vi "TL_Driver.vi"(0 "Device In":refnum<visa-resource-name>="Pro8000", 5 "Commands":T1(ring)=enum."SET", 7 "Settings":T3={"Module"=enum."Off Line TEC", "OnLineTEC"=23.2280006, "OnLineLD"=0.1722, "OffLineTEC"=29.538, "OffLineLD"=0.173, "EtalonTEC"=27.0004501, "TSOA-TEC"=18.9999638} {"OffLineLD" min=0.0 max=0.18 step=0.001 format="%.3p"; "OnLineLD" min=0.0 max=0.18 step=0.001 format="%.3p"; "TSOA-TEC" format="%.2g"; "EtalonTEC" format="%.2g"; "OffLineTEC" min=16.0 max=30.0 step=0.1 format="%.3g"; "OnLineTEC" min=16.0 max=28.0 step=0.1 format="%.3g"}, 11 "error in":errorcluster) -> (4 "Device Out":refnum<visa-resource-name>="Pro8000", 6 "Response":string, 8 "Readings":T2={"OnLineTEC"=23.2342777, "OnLineLD"=0.172234386, "OffLineTEC"=29.5498905, "OffLineLD"=0.17301172, "EtalonTEC"=27.0301247, "TSOA-TEC"=19.0111637, "Pro8000"=TRUE, "OnLine TEC"=TRUE, "OnLine LD"=TRUE, "OffLine TEC"=TRUE, "OffLine LD"=TRUE, "Etalon TEC"=TRUE, "TSOA TEC"=TRUE} {"OffLineLD" format="%.3p"; "OnLineLD" format="%.3p"; "TSOA-TEC" format="%.3g"; "EtalonTEC" format="%.3g"; "OffLineTEC" format="%.3g"; "OnLineTEC" format="%.3g"}, 15 "error out":errorcluster)   [LabVIEW 2012]
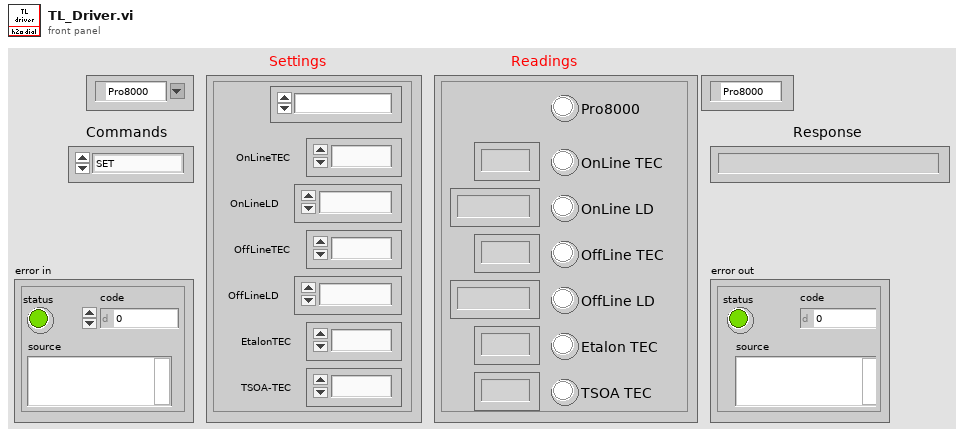
[diagram p1: front panel]
types:
  T1 = enum16{"Open_TL", "Close_TL", "Verify_ID", "TEC_Sensor", "SET", "READ", "ON", "OFF", "Set_Limits", "Read_Limits", "Enable_Status", "Read_Status"}
  T2 = cluster{"OnLineTEC":dbl, "OnLineLD":dbl, "OffLineTEC":dbl, "OffLineLD":dbl, "EtalonTEC":dbl, "TSOA-TEC":dbl, "Pro8000":bool, "OnLine TEC":bool, "OnLine LD":bool, "OffLine TEC":bool, "OffLine LD":bool, "Etalon TEC":bool, "TSOA TEC":bool}
  T3 = cluster{"Module":enum16{"On Line TEC", "On Line LD", "Off Line TEC", "Off Line LD", "Etalon TEC", "TSOA TEC"}, "OnLineTEC":dbl, "OnLineLD":dbl, "OffLineTEC":dbl, "OffLineLD":dbl, "EtalonTEC":dbl, "TSOA-TEC":dbl}
  T4 = enum16{"On Line TEC", "On Line LD", "Off Line TEC", "Off Line LD", "Etalon TEC", "TSOA TEC"}
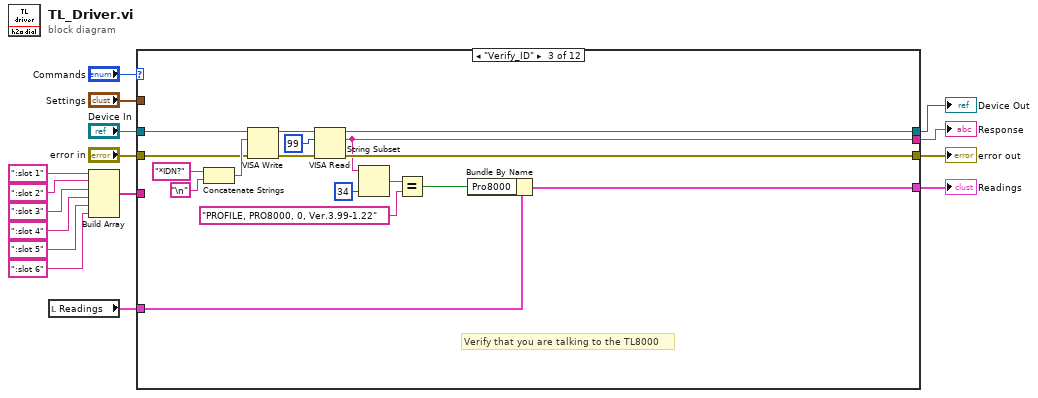
[diagram p0: block diagram]
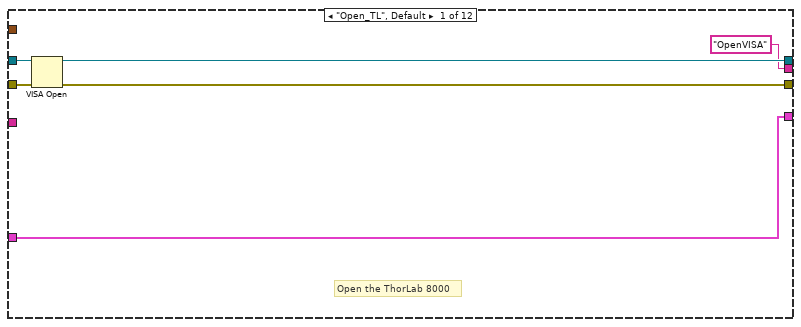
[diagram p2: hidden frame]
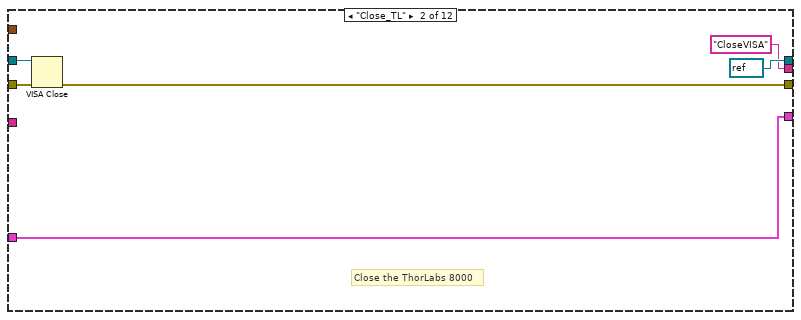
[diagram p3: hidden frame]
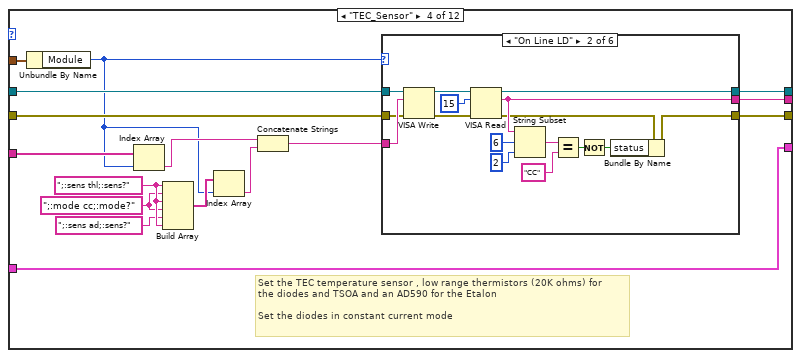
[diagram p4: hidden frame]
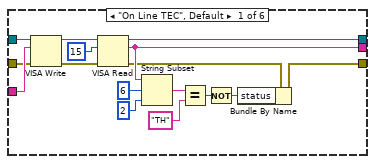
[diagram p5: hidden frame]
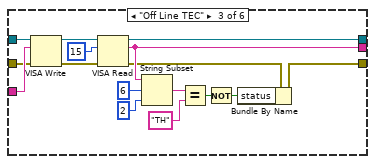
[diagram p6: hidden frame]
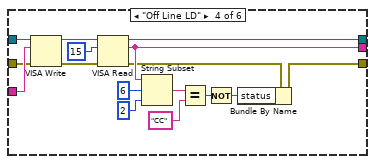
[diagram p7: hidden frame]
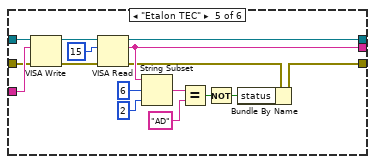
[diagram p8: hidden frame]
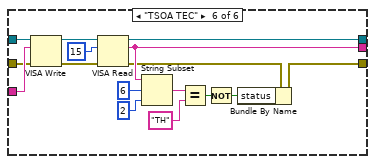
[diagram p9: hidden frame]
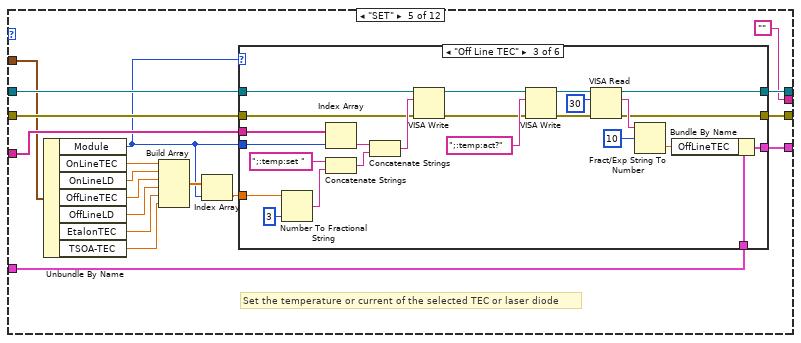
[diagram p10: hidden frame]
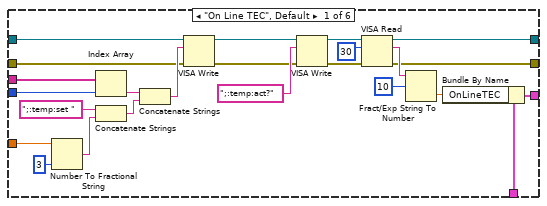
[diagram p11: hidden frame]
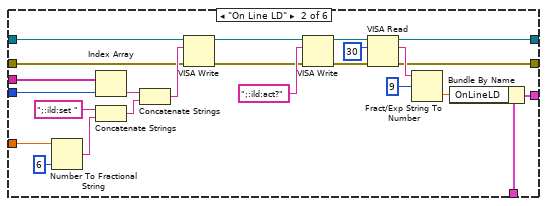
[diagram p12: hidden frame]
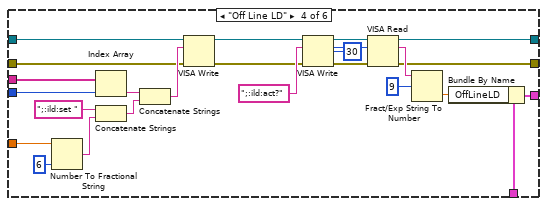
[diagram p13: hidden frame]
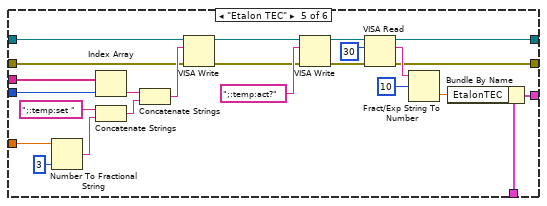
[diagram p14: hidden frame]
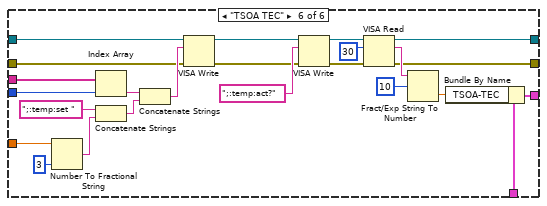
[diagram p15: hidden frame]
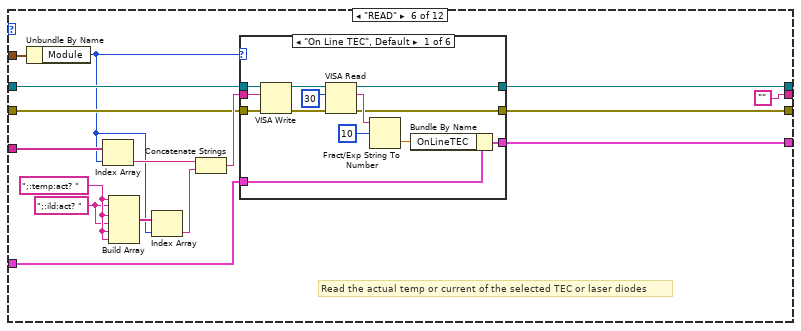
[diagram p16: hidden frame]
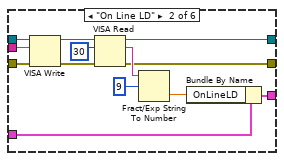
[diagram p17: hidden frame]
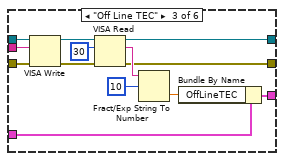
[diagram p18: hidden frame]
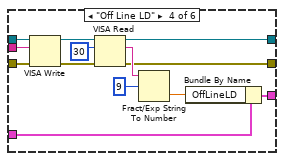
[diagram p19: hidden frame]
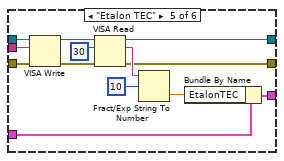
[diagram p20: hidden frame]
diagram:
  n1 = local read "Readings"() -> (w2:T2)
  n2 = Build Array(":slot 1", ":slot 2", ":slot 3", ":slot 4", ":slot 5", ":slot 6") -> (w13:string[])
  n3 = case shown="\"Verify_ID\"" "Commands" {
    tunnel: "Device In" -> [w22 w28 w42 w60 w175 w334 w428 w552 w668 w672 w676 w683]
    tunnel: "error in" -> [w21 w27 w39 w59 w174 w333 w427 w551 w669 w673 w677 w686]
    tunnel: [w20 refnum<visa-resource-name> refnum ("VISA resource name") w37 w58 w171 w329 w424 w548 w668 w672 w676 w684] -> w11
    tunnel: [w19 w26 w36 w55 w172 w328 w423 w547 w669 w673 w677 w682] -> w15
    tunnel: ["OpenVISA" "CloseVISA" w35 w57 "" "" w422 w546 "" "" "" "Read Status"] -> w10
    tunnel: w13 -> [_ _ _ w54 w173 w331 w425 w549 _ _ _ w687]
    tunnel: "Settings" -> [_ _ _ w53 w169 w327 w421 w545 _ _ _ w685]
    tunnel: w2 -> [w17 w23 w31 w47 w159 w326 w420 w544 w670 w674 w678 w681]
    tunnel: [w17 w23 w30 w47 w158 w325 w419 w543 w670 w674 w678 w680] -> w1
    frame "Open_TL", Default {
      # "Open the ThorLab 8000"
      n4 = VISA Open(error in (no error)=w21, VISA resource name=w22) -> (VISA resource name=w20:refnum<visa-resource-name>, error out=w19:errorcluster)  [unwired: 3 in]
    }
    frame "Close_TL" {
      # "Close the ThorLabs 8000"
      n5 = VISA Close(VISA resource name=w28, error in (no error)=w27) -> (error out=w26:errorcluster)
    }
    frame "Verify_ID" {
      # "Verify that you are talking to the TL8000"
      n6 = Concatenate Strings("*IDN?" ("string"), "\n") -> (w43:string)
      n7 = VISA Write(VISA resource name=w42, write buffer=w43, error in (no error)=w39) -> (VISA resource name out=w40:refnum<visa-resource-name>, error out=w38:errorcluster)  [unwired: 1 out]
      n8 = VISA Read(VISA resource name=w40, byte count=u32 99, error in (no error)=w38) -> (VISA resource name out=w37:refnum<visa-resource-name>, read buffer=w35:string, error out=w36:errorcluster)  [unwired: 1 out]
      n9 = String Subset(string=w35, length (rest)=34 ("length (rest)")) -> (substring=w33:string)  [unwired: 1 in]
      n10 = Equal?(x=w33, y="PROFILE, PRO8000, 0, Ver.3.99-1.22" ("Response")) -> (x = y?=w29:bool)
      n11 = Bundle By Name(cluster=w31, "Pro8000"=w29) -> (w30:T2)
    }
    frame "TEC_Sensor" {
      w46 = ";:mode cc;:mode?"
      w52 = ";:sens thl;:sens?" ("string")
      # "Set the TEC temperature sensor , low range thermistors (20K ohms) for\nthe diodes and TSOA and an AD590 for the Etalon\n\nSet the diodes in constant current mode"
      n12 = Unbundle By Name(w53) -> ("Module"=w48:T4)
      n13 = Index Array(array=w54, index=w48) -> (element=w56:string)
      n14 = Build Array(w52, w46, w52, w46, ";:sens ad;:sens?" ("string"), w52) -> (w49:string[])
      n15 = Index Array(array=w49, index=w48) -> (element=w50:string)
      n16 = Concatenate Strings(w56, w50) -> (w61:string)
      n17 = case shown="\"On Line LD\"" w48 {
        tunnel: w61 -> [w77 w93 w109 w125 w141 w157]
        tunnel: w60 -> [w76 w92 w108 w124 w140 w156]
        tunnel: w59 -> [w75 w91 w107 w123 w139 w155]
        tunnel: [w74 w90 w106 w122 w138 w154] -> w58
        tunnel: [w73 w89 w105 w121 w137 w153] -> w57
        tunnel: [w72 w88 w104 w120 w136 w152] -> w55
        frame "On Line TEC", Default {
          n18 = VISA Write(VISA resource name=w76, write buffer=w77, error in (no error)=w75) -> (VISA resource name out=w64:refnum<visa-resource-name>, error out=w63:errorcluster)  [unwired: 1 out]
          n19 = VISA Read(VISA resource name=w64, byte count=u32 15, error in (no error)=w63) -> (VISA resource name out=w74:refnum<visa-resource-name>, read buffer=w73:string, error out=w70:errorcluster)  [unwired: 1 out]
          n20 = String Subset(string=w73, offset (0)=6 ("length (rest)"), length (rest)=2 ("length (rest)")) -> (substring=w67:string)
          n21 = Equal?(x=w67, y="TH") -> (x = y?=w66:bool)
          n22 = Not(x=w66) -> (.not. x?=w65:bool)
          n23 = Bundle By Name(cluster=w70, "status"=w65) -> (w72:errorcluster)
        }
        frame "On Line LD" {
          n24 = VISA Write(VISA resource name=w92, write buffer=w93, error in (no error)=w91) -> (VISA resource name out=w80:refnum<visa-resource-name>, error out=w79:errorcluster)  [unwired: 1 out]
          n25 = VISA Read(VISA resource name=w80, byte count=u32 15, error in (no error)=w79) -> (VISA resource name out=w90:refnum<visa-resource-name>, read buffer=w89:string, error out=w86:errorcluster)  [unwired: 1 out]
          n26 = String Subset(string=w89, offset (0)=6 ("length (rest)"), length (rest)=2 ("length (rest)")) -> (substring=w83:string)
          n27 = Equal?(x=w83, y="CC") -> (x = y?=w82:bool)
          n28 = Not(x=w82) -> (.not. x?=w81:bool)
          n29 = Bundle By Name(cluster=w86, "status"=w81) -> (w88:errorcluster)
        }
        frame "Off Line TEC" {
          n30 = VISA Write(VISA resource name=w108, write buffer=w109, error in (no error)=w107) -> (VISA resource name out=w96:refnum<visa-resource-name>, error out=w95:errorcluster)  [unwired: 1 out]
          n31 = VISA Read(VISA resource name=w96, byte count=u32 15, error in (no error)=w95) -> (VISA resource name out=w106:refnum<visa-resource-name>, read buffer=w105:string, error out=w102:errorcluster)  [unwired: 1 out]
          n32 = String Subset(string=w105, offset (0)=6 ("length (rest)"), length (rest)=2 ("length (rest)")) -> (substring=w99:string)
          n33 = Equal?(x=w99, y="TH") -> (x = y?=w98:bool)
          n34 = Not(x=w98) -> (.not. x?=w97:bool)
          n35 = Bundle By Name(cluster=w102, "status"=w97) -> (w104:errorcluster)
        }
        frame "Off Line LD" {
          n36 = VISA Write(VISA resource name=w124, write buffer=w125, error in (no error)=w123) -> (VISA resource name out=w112:refnum<visa-resource-name>, error out=w111:errorcluster)  [unwired: 1 out]
          n37 = VISA Read(VISA resource name=w112, byte count=u32 15, error in (no error)=w111) -> (VISA resource name out=w122:refnum<visa-resource-name>, read buffer=w121:string, error out=w118:errorcluster)  [unwired: 1 out]
          n38 = String Subset(string=w121, offset (0)=6 ("length (rest)"), length (rest)=2 ("length (rest)")) -> (substring=w115:string)
          n39 = Equal?(x=w115, y="CC") -> (x = y?=w114:bool)
          n40 = Not(x=w114) -> (.not. x?=w113:bool)
          n41 = Bundle By Name(cluster=w118, "status"=w113) -> (w120:errorcluster)
        }
        frame "Etalon TEC" {
          n42 = VISA Write(VISA resource name=w140, write buffer=w141, error in (no error)=w139) -> (VISA resource name out=w128:refnum<visa-resource-name>, error out=w127:errorcluster)  [unwired: 1 out]
          n43 = VISA Read(VISA resource name=w128, byte count=u32 15, error in (no error)=w127) -> (VISA resource name out=w138:refnum<visa-resource-name>, read buffer=w137:string, error out=w134:errorcluster)  [unwired: 1 out]
          n44 = String Subset(string=w137, offset (0)=6 ("length (rest)"), length (rest)=2 ("length (rest)")) -> (substring=w131:string)
          n45 = Equal?(x=w131, y="AD") -> (x = y?=w130:bool)
          n46 = Not(x=w130) -> (.not. x?=w129:bool)
          n47 = Bundle By Name(cluster=w134, "status"=w129) -> (w136:errorcluster)
        }
        frame "TSOA TEC" {
          n48 = VISA Write(VISA resource name=w156, write buffer=w157, error in (no error)=w155) -> (VISA resource name out=w144:refnum<visa-resource-name>, error out=w143:errorcluster)  [unwired: 1 out]
          n49 = VISA Read(VISA resource name=w144, byte count=u32 15, error in (no error)=w143) -> (VISA resource name out=w154:refnum<visa-resource-name>, read buffer=w153:string, error out=w150:errorcluster)  [unwired: 1 out]
          n50 = String Subset(string=w153, offset (0)=6 ("length (rest)"), length (rest)=2 ("length (rest)")) -> (substring=w147:string)
          n51 = Equal?(x=w147, y="TH") -> (x = y?=w146:bool)
          n52 = Not(x=w146) -> (.not. x?=w145:bool)
          n53 = Bundle By Name(cluster=w150, "status"=w145) -> (w152:errorcluster)
        }
      }
    }
    frame "SET" {
      # "Set the temperature or current of the selected TEC or laser diode"
      n54 = Unbundle By Name(w169) -> ("Module"=w166:T4, "OnLineTEC"=w165:dbl, "OnLineLD"=w164:dbl, "OffLineTEC"=w163:dbl, "OffLineLD"=w162:dbl, "EtalonTEC"=w161:dbl, "TSOA-TEC"=w160:dbl)
      n55 = Build Array(w165, w164, w163, w162, w161, w160) -> (w168:dbl[])
      n56 = Index Array(array=w168, index=w166) -> (element=w167:dbl)
      n57 = case shown="\"Off Line TEC\"" w166 {
        tunnel: w175 -> [w198 w222 w246 w270 w294 w318]
        tunnel: w174 -> [w197 w221 w245 w269 w293 w317]
        tunnel: w173 -> [w195 w219 w243 w267 w291 w315]
        tunnel: [w180 w206 w228 w253 w276 w299] -> w172
        tunnel: [w179 w205 w226 w252 w275 w298] -> w171
        tunnel: w167 -> [w189 w213 w237 w261 w285 w309]
        tunnel: w166 -> [w190 w214 w238 w262 w286 w310]
        tunnel: w159 -> [w182 w203 w230 w251 w277 w301]
        tunnel: [w181 w202 w229 w250 w278 w302] -> w158
        frame "On Line TEC", Default {
          n58 = Number To Fractional String(number=w189, precision (6)=i16 3) -> (F-format string=w194:string)  [unwired: 2 in]
          n59 = Index Array(array=w195, index=w190) -> (element=w196:string)
          n60 = Concatenate Strings(";:temp:set " ("write buffer"), w194) -> (w191:string)
          n61 = Concatenate Strings(w196, w191) -> (w199:string)
          n62 = VISA Write(VISA resource name=w198, write buffer=w199, error in (no error)=w197) -> (VISA resource name out=w177:refnum<visa-resource-name>, error out=w176:errorcluster)  [unwired: 1 out]
          n63 = VISA Write(VISA resource name=w177, write buffer=";:temp:act?", error in (no error)=w176) -> (VISA resource name out=w184:refnum<visa-resource-name>, error out=w185:errorcluster)  [unwired: 1 out]
          n64 = VISA Read(VISA resource name=w184, byte count=u32 30, error in (no error)=w185) -> (VISA resource name out=w179:refnum<visa-resource-name>, read buffer=w186:string, error out=w180:errorcluster)  [unwired: 1 out]
          n65 = Fract/Exp String To Number(string=w186, offset=10) -> (number=w183:dbl)  [unwired: 2 in, 1 out]
          n66 = Bundle By Name(cluster=w182, "OnLineTEC"=w183) -> (w181:T2)
        }
        frame "On Line LD" {
          n67 = Number To Fractional String(number=w213, precision (6)=i16 6) -> (F-format string=w218:string)  [unwired: 2 in]
          n68 = Index Array(array=w219, index=w214) -> (element=w220:string)
          n69 = Concatenate Strings(";:ild:set " ("write buffer"), w218) -> (w215:string)
          n70 = Concatenate Strings(w220, w215) -> (w223:string)
          n71 = VISA Write(VISA resource name=w222, write buffer=w223, error in (no error)=w221) -> (VISA resource name out=w201:refnum<visa-resource-name>, error out=w200:errorcluster)  [unwired: 1 out]
          n72 = VISA Write(VISA resource name=w201, write buffer=";:ild:act?", error in (no error)=w200) -> (VISA resource name out=w208:refnum<visa-resource-name>, error out=w209:errorcluster)  [unwired: 1 out]
          n73 = VISA Read(VISA resource name=w208, byte count=u32 30, error in (no error)=w209) -> (VISA resource name out=w205:refnum<visa-resource-name>, read buffer=w210:string, error out=w206:errorcluster)  [unwired: 1 out]
          n74 = Fract/Exp String To Number(string=w210, offset=9) -> (number=w207:dbl)  [unwired: 2 in, 1 out]
          n75 = Bundle By Name(cluster=w203, "OnLineLD"=w207) -> (w202:T2)
        }
        frame "Off Line TEC" {
          n76 = Number To Fractional String(number=w237, precision (6)=i16 3) -> (F-format string=w242:string)  [unwired: 2 in]
          n77 = Index Array(array=w243, index=w238) -> (element=w244:string)
          n78 = Concatenate Strings(";:temp:set " ("write buffer"), w242) -> (w239:string)
          n79 = Concatenate Strings(w244, w239) -> (w247:string)
          n80 = VISA Write(VISA resource name=w246, write buffer=w247, error in (no error)=w245) -> (VISA resource name out=w225:refnum<visa-resource-name>, error out=w224:errorcluster)  [unwired: 1 out]
          n81 = VISA Write(VISA resource name=w225, write buffer=";:temp:act?", error in (no error)=w224) -> (VISA resource name out=w227:refnum<visa-resource-name>, error out=w233:errorcluster)  [unwired: 1 out]
          n82 = VISA Read(VISA resource name=w227, byte count=u32 30, error in (no error)=w233) -> (VISA resource name out=w226:refnum<visa-resource-name>, read buffer=w234:string, error out=w228:errorcluster)  [unwired: 1 out]
          n83 = Fract/Exp String To Number(string=w234, offset=10) -> (number=w232:dbl)  [unwired: 2 in, 1 out]
          n84 = Bundle By Name(cluster=w230, "OffLineTEC"=w232) -> (w229:T2)
        }
        frame "Off Line LD" {
          n85 = Number To Fractional String(number=w261, precision (6)=i16 6) -> (F-format string=w266:string)  [unwired: 2 in]
          n86 = Index Array(array=w267, index=w262) -> (element=w268:string)
          n87 = Concatenate Strings(";:ild:set " ("write buffer"), w266) -> (w263:string)
          n88 = Concatenate Strings(w268, w263) -> (w271:string)
          n89 = VISA Write(VISA resource name=w270, write buffer=w271, error in (no error)=w269) -> (VISA resource name out=w249:refnum<visa-resource-name>, error out=w248:errorcluster)  [unwired: 1 out]
          n90 = VISA Write(VISA resource name=w249, write buffer=";:ild:act?", error in (no error)=w248) -> (VISA resource name out=w256:refnum<visa-resource-name>, error out=w257:errorcluster)  [unwired: 1 out]
          n91 = VISA Read(VISA resource name=w256, byte count=u32 30, error in (no error)=w257) -> (VISA resource name out=w252:refnum<visa-resource-name>, read buffer=w258:string, error out=w253:errorcluster)  [unwired: 1 out]
          n92 = Fract/Exp String To Number(string=w258, offset=9) -> (number=w255:dbl)  [unwired: 2 in, 1 out]
          n93 = Bundle By Name(cluster=w251, "OffLineLD"=w255) -> (w250:T2)
        }
        frame "Etalon TEC" {
          n94 = Number To Fractional String(number=w285, precision (6)=i16 3) -> (F-format string=w290:string)  [unwired: 2 in]
          n95 = Index Array(array=w291, index=w286) -> (element=w292:string)
          n96 = Concatenate Strings(";:temp:set " ("write buffer"), w290) -> (w287:string)
          n97 = Concatenate Strings(w292, w287) -> (w295:string)
          n98 = VISA Write(VISA resource name=w294, write buffer=w295, error in (no error)=w293) -> (VISA resource name out=w273:refnum<visa-resource-name>, error out=w272:errorcluster)  [unwired: 1 out]
          n99 = VISA Write(VISA resource name=w273, write buffer=";:temp:act?", error in (no error)=w272) -> (VISA resource name out=w274:refnum<visa-resource-name>, error out=w281:errorcluster)  [unwired: 1 out]
          n100 = VISA Read(VISA resource name=w274, byte count=u32 30, error in (no error)=w281) -> (VISA resource name out=w275:refnum<visa-resource-name>, read buffer=w282:string, error out=w276:errorcluster)  [unwired: 1 out]
          n101 = Fract/Exp String To Number(string=w282, offset=10) -> (number=w280:dbl)  [unwired: 2 in, 1 out]
          n102 = Bundle By Name(cluster=w277, "EtalonTEC"=w280) -> (w278:T2)
        }
        frame "TSOA TEC" {
          n103 = Number To Fractional String(number=w309, precision (6)=i16 3) -> (F-format string=w314:string)  [unwired: 2 in]
          n104 = Index Array(array=w315, index=w310) -> (element=w316:string)
          n105 = Concatenate Strings(";:temp:set " ("write buffer"), w314) -> (w311:string)
          n106 = Concatenate Strings(w316, w311) -> (w319:string)
          n107 = VISA Write(VISA resource name=w318, write buffer=w319, error in (no error)=w317) -> (VISA resource name out=w297:refnum<visa-resource-name>, error out=w296:errorcluster)  [unwired: 1 out]
          n108 = VISA Write(VISA resource name=w297, write buffer=";:temp:act?", error in (no error)=w296) -> (VISA resource name out=w300:refnum<visa-resource-name>, error out=w305:errorcluster)  [unwired: 1 out]
          n109 = VISA Read(VISA resource name=w300, byte count=u32 30, error in (no error)=w305) -> (VISA resource name out=w298:refnum<visa-resource-name>, read buffer=w306:string, error out=w299:errorcluster)  [unwired: 1 out]
          n110 = Fract/Exp String To Number(string=w306, offset=10) -> (number=w304:dbl)  [unwired: 2 in, 1 out]
          n111 = Bundle By Name(cluster=w301, "TSOA-TEC"=w304) -> (w302:T2)
        }
      }
    }
    frame "READ" {
      w323 = ";:ild:act? " ("write buffer")
      w324 = ";:temp:act? " ("write buffer")
      # "Read the actual temp or current of the selected TEC or laser diodes"
      n112 = Unbundle By Name(w327) -> ("Module"=w321:T4)
      n113 = Index Array(array=w331, index=w321) -> (element=w332:string)
      n114 = Build Array(w324, w323, w324, w323, w324, w324) -> (w322:string[])
      n115 = Index Array(array=w322, index=w321) -> (element=w320:string)
      n116 = Concatenate Strings(w332, w320) -> (w335:string)
      n117 = case shown="\"On Line TEC\", Default" w321 {
        tunnel: w335 -> [w348 w361 w374 w387 w400 w413]
        tunnel: w334 -> [w347 w360 w373 w386 w399 w412]
        tunnel: w333 -> [w346 w359 w372 w385 w398 w411]
        tunnel: [w340 w353 w366 w379 w392 w405] -> w329
        tunnel: [w339 w352 w365 w378 w391 w404] -> w328
        tunnel: w326 -> [w337 w350 w363 w376 w389 w402]
        tunnel: [w336 w349 w362 w375 w388 w401] -> w325
        frame "On Line TEC", Default {
          n118 = VISA Write(VISA resource name=w347, write buffer=w348, error in (no error)=w346) -> (VISA resource name out=w341:refnum<visa-resource-name>, error out=w342:errorcluster)  [unwired: 1 out]
          n119 = VISA Read(VISA resource name=w341, byte count=u32 30, error in (no error)=w342) -> (VISA resource name out=w340:refnum<visa-resource-name>, read buffer=w343:string, error out=w339:errorcluster)  [unwired: 1 out]
          n120 = Fract/Exp String To Number(string=w343, offset=10) -> (number=w338:dbl)  [unwired: 2 in, 1 out]
          n121 = Bundle By Name(cluster=w337, "OnLineTEC"=w338) -> (w336:T2)
        }
        frame "On Line LD" {
          n122 = VISA Write(VISA resource name=w360, write buffer=w361, error in (no error)=w359) -> (VISA resource name out=w354:refnum<visa-resource-name>, error out=w355:errorcluster)  [unwired: 1 out]
          n123 = VISA Read(VISA resource name=w354, byte count=u32 30, error in (no error)=w355) -> (VISA resource name out=w353:refnum<visa-resource-name>, read buffer=w356:string, error out=w352:errorcluster)  [unwired: 1 out]
          n124 = Fract/Exp String To Number(string=w356, offset=9) -> (number=w351:dbl)  [unwired: 2 in, 1 out]
          n125 = Bundle By Name(cluster=w350, "OnLineLD"=w351) -> (w349:T2)
        }
        frame "Off Line TEC" {
          n126 = VISA Write(VISA resource name=w373, write buffer=w374, error in (no error)=w372) -> (VISA resource name out=w367:refnum<visa-resource-name>, error out=w368:errorcluster)  [unwired: 1 out]
          n127 = VISA Read(VISA resource name=w367, byte count=u32 30, error in (no error)=w368) -> (VISA resource name out=w366:refnum<visa-resource-name>, read buffer=w369:string, error out=w365:errorcluster)  [unwired: 1 out]
          n128 = Fract/Exp String To Number(string=w369, offset=10) -> (number=w364:dbl)  [unwired: 2 in, 1 out]
          n129 = Bundle By Name(cluster=w363, "OffLineTEC"=w364) -> (w362:T2)
        }
        frame "Off Line LD" {
          n130 = VISA Write(VISA resource name=w386, write buffer=w387, error in (no error)=w385) -> (VISA resource name out=w380:refnum<visa-resource-name>, error out=w381:errorcluster)  [unwired: 1 out]
          n131 = VISA Read(VISA resource name=w380, byte count=u32 30, error in (no error)=w381) -> (VISA resource name out=w379:refnum<visa-resource-name>, read buffer=w382:string, error out=w378:errorcluster)  [unwired: 1 out]
          n132 = Fract/Exp String To Number(string=w382, offset=9) -> (number=w377:dbl)  [unwired: 2 in, 1 out]
          n133 = Bundle By Name(cluster=w376, "OffLineLD"=w377) -> (w375:T2)
        }
        frame "Etalon TEC" {
          n134 = VISA Write(VISA resource name=w399, write buffer=w400, error in (no error)=w398) -> (VISA resource name out=w393:refnum<visa-resource-name>, error out=w394:errorcluster)  [unwired: 1 out]
          n135 = VISA Read(VISA resource name=w393, byte count=u32 30, error in (no error)=w394) -> (VISA resource name out=w392:refnum<visa-resource-name>, read buffer=w395:string, error out=w391:errorcluster)  [unwired: 1 out]
          n136 = Fract/Exp String To Number(string=w395, offset=10) -> (number=w390:dbl)  [unwired: 2 in, 1 out]
          n137 = Bundle By Name(cluster=w389, "EtalonTEC"=w390) -> (w388:T2)
        }
        frame "TSOA TEC" {
          n138 = VISA Write(VISA resource name=w412, write buffer=w413, error in (no error)=w411) -> (VISA resource name out=w406:refnum<visa-resource-name>, error out=w407:errorcluster)  [unwired: 1 out]
          n139 = VISA Read(VISA resource name=w406, byte count=u32 30, error in (no error)=w407) -> (VISA resource name out=w405:refnum<visa-resource-name>, read buffer=w408:string, error out=w404:errorcluster)  [unwired: 1 out]
          n140 = Fract/Exp String To Number(string=w408, offset=10) -> (number=w403:dbl)  [unwired: 2 in, 1 out]
          n141 = Bundle By Name(cluster=w402, "TSOA-TEC"=w403) -> (w401:T2)
        }
      }
    }
    frame "ON" {
      w418 = ";:laser on" ("write buffer")
      w416 = ";:tec on" ("write buffer")
      # "Turn the selected TEC or laser on"
      n142 = Unbundle By Name(w421) -> ("Module"=w415:T4)
      n143 = Build Array(w416, w418, w416, w418, w416, w416) -> (w417:string[])
      n144 = Index Array(array=w425, index=w415) -> (element=w426:string)
      n145 = Index Array(array=w417, index=w415) -> (element=w414:string)
      n146 = Concatenate Strings(w426, w414) -> (w429:string)
      n147 = case shown="\"On Line TEC\", Default" w415 {
        tunnel: w429 -> [w447 w465 w483 w501 w519 w537]
        tunnel: w428 -> [w446 w464 w482 w500 w518 w536]
        tunnel: w427 -> [w445 w463 w481 w499 w517 w535]
        tunnel: [w443 w461 w479 w497 w515 w533] -> w424
        tunnel: [w442 w460 w478 w496 w514 w532] -> w423
        tunnel: [w433 w451 w469 w487 w505 w523] -> w422
        tunnel: w420 -> [w432 w450 w468 w486 w504 w522]
        tunnel: [w431 w449 w467 w485 w503 w521] -> w419
        frame "On Line TEC", Default {
          n148 = VISA Write(VISA resource name=w446, write buffer=w447, error in (no error)=w445) -> (VISA resource name out=w439:refnum<visa-resource-name>, error out=w441:errorcluster)  [unwired: 1 out]
          n149 = VISA Write(VISA resource name=w439, write buffer=":tec?", error in (no error)=w441) -> (VISA resource name out=w438:refnum<visa-resource-name>, error out=w440:errorcluster)  [unwired: 1 out]
          n150 = VISA Read(VISA resource name=w438, byte count=u32 15, error in (no error)=w440) -> (VISA resource name out=w443:refnum<visa-resource-name>, read buffer=w433:string, error out=w442:errorcluster)  [unwired: 1 out]
          n151 = String Subset(string=w433, length (rest)=7 ("offset (0)")) -> (substring=w435:string)  [unwired: 1 in]
          n152 = Equal?(x=w435, y=":TEC ON") -> (x = y?=w430:bool)
          n153 = Bundle By Name(cluster=w432, "OnLine TEC"=w430) -> (w431:T2)
        }
        frame "On Line LD" {
          n154 = VISA Write(VISA resource name=w464, write buffer=w465, error in (no error)=w463) -> (VISA resource name out=w457:refnum<visa-resource-name>, error out=w459:errorcluster)  [unwired: 1 out]
          n155 = VISA Write(VISA resource name=w457, write buffer=":laser?", error in (no error)=w459) -> (VISA resource name out=w456:refnum<visa-resource-name>, error out=w458:errorcluster)  [unwired: 1 out]
          n156 = VISA Read(VISA resource name=w456, byte count=u32 15, error in (no error)=w458) -> (VISA resource name out=w461:refnum<visa-resource-name>, read buffer=w451:string, error out=w460:errorcluster)  [unwired: 1 out]
          n157 = String Subset(string=w451, length (rest)=9 ("offset (0)")) -> (substring=w453:string)  [unwired: 1 in]
          n158 = Equal?(x=w453, y=":LASER ON") -> (x = y?=w448:bool)
          n159 = Bundle By Name(cluster=w450, "OnLine LD"=w448) -> (w449:T2)
        }
        frame "Off Line TEC" {
          n160 = VISA Write(VISA resource name=w482, write buffer=w483, error in (no error)=w481) -> (VISA resource name out=w475:refnum<visa-resource-name>, error out=w477:errorcluster)  [unwired: 1 out]
          n161 = VISA Write(VISA resource name=w475, write buffer=":tec?", error in (no error)=w477) -> (VISA resource name out=w474:refnum<visa-resource-name>, error out=w476:errorcluster)  [unwired: 1 out]
          n162 = VISA Read(VISA resource name=w474, byte count=u32 15, error in (no error)=w476) -> (VISA resource name out=w479:refnum<visa-resource-name>, read buffer=w469:string, error out=w478:errorcluster)  [unwired: 1 out]
          n163 = String Subset(string=w469, length (rest)=7 ("offset (0)")) -> (substring=w471:string)  [unwired: 1 in]
          n164 = Equal?(x=w471, y=":TEC ON") -> (x = y?=w466:bool)
          n165 = Bundle By Name(cluster=w468, "OffLine TEC"=w466) -> (w467:T2)
        }
        frame "Off Line LD" {
          n166 = VISA Write(VISA resource name=w500, write buffer=w501, error in (no error)=w499) -> (VISA resource name out=w493:refnum<visa-resource-name>, error out=w495:errorcluster)  [unwired: 1 out]
          n167 = VISA Write(VISA resource name=w493, write buffer=":laser?", error in (no error)=w495) -> (VISA resource name out=w492:refnum<visa-resource-name>, error out=w494:errorcluster)  [unwired: 1 out]
          n168 = VISA Read(VISA resource name=w492, byte count=u32 15, error in (no error)=w494) -> (VISA resource name out=w497:refnum<visa-resource-name>, read buffer=w487:string, error out=w496:errorcluster)  [unwired: 1 out]
          n169 = String Subset(string=w487, length (rest)=9 ("offset (0)")) -> (substring=w489:string)  [unwired: 1 in]
          n170 = Equal?(x=w489, y=":LASER ON") -> (x = y?=w484:bool)
          n171 = Bundle By Name(cluster=w486, "OffLine LD"=w484) -> (w485:T2)
        }
        frame "Etalon TEC" {
          n172 = VISA Write(VISA resource name=w518, write buffer=w519, error in (no error)=w517) -> (VISA resource name out=w511:refnum<visa-resource-name>, error out=w513:errorcluster)  [unwired: 1 out]
          n173 = VISA Write(VISA resource name=w511, write buffer=":tec?", error in (no error)=w513) -> (VISA resource name out=w510:refnum<visa-resource-name>, error out=w512:errorcluster)  [unwired: 1 out]
          n174 = VISA Read(VISA resource name=w510, byte count=u32 15, error in (no error)=w512) -> (VISA resource name out=w515:refnum<visa-resource-name>, read buffer=w505:string, error out=w514:errorcluster)  [unwired: 1 out]
          n175 = String Subset(string=w505, length (rest)=7 ("offset (0)")) -> (substring=w507:string)  [unwired: 1 in]
          n176 = Equal?(x=w507, y=":TEC ON") -> (x = y?=w502:bool)
          n177 = Bundle By Name(cluster=w504, "Etalon TEC"=w502) -> (w503:T2)
        }
        frame "TSOA TEC" {
          n178 = VISA Write(VISA resource name=w536, write buffer=w537, error in (no error)=w535) -> (VISA resource name out=w529:refnum<visa-resource-name>, error out=w531:errorcluster)  [unwired: 1 out]
          n179 = VISA Write(VISA resource name=w529, write buffer=":tec?", error in (no error)=w531) -> (VISA resource name out=w528:refnum<visa-resource-name>, error out=w530:errorcluster)  [unwired: 1 out]
          n180 = VISA Read(VISA resource name=w528, byte count=u32 15, error in (no error)=w530) -> (VISA resource name out=w533:refnum<visa-resource-name>, read buffer=w523:string, error out=w532:errorcluster)  [unwired: 1 out]
          n181 = String Subset(string=w523, length (rest)=7 ("offset (0)")) -> (substring=w525:string)  [unwired: 1 in]
          n182 = Equal?(x=w525, y=":TEC ON") -> (x = y?=w520:bool)
          n183 = Bundle By Name(cluster=w522, "TSOA TEC"=w520) -> (w521:T2)
        }
      }
    }
    frame "OFF" {
      w541 = ";:laser off" ("write buffer")
      w542 = ";:tec off" ("write buffer")
      # "Turn the selected TEC or laser off"
      n184 = Unbundle By Name(w545) -> ("Module"=w538:T4)
      n185 = Build Array(w542, w541, w542, w541, w542, w542) -> (w540:string[])
      n186 = Index Array(array=w549, index=w538) -> (element=w550:string)
      n187 = Index Array(array=w540, index=w538) -> (element=w539:string)
      n188 = Concatenate Strings(w550, w539) -> (w553:string)
      n189 = case shown="\"On Line TEC\", Default" w538 {
        tunnel: w553 -> [w572 w591 w610 w629 w648 w667]
        tunnel: w552 -> [w571 w590 w609 w628 w647 w666]
        tunnel: w551 -> [w570 w589 w608 w627 w646 w665]
        tunnel: [w568 w587 w606 w625 w644 w663] -> w548
        tunnel: [w567 w586 w605 w624 w643 w662] -> w547
        tunnel: [w558 w577 w596 w615 w634 w653] -> w546
        tunnel: w544 -> [w557 w576 w595 w614 w633 w652]
        tunnel: [w556 w575 w594 w613 w632 w651] -> w543
        frame "On Line TEC", Default {
          n190 = VISA Write(VISA resource name=w571, write buffer=w572, error in (no error)=w570) -> (VISA resource name out=w564:refnum<visa-resource-name>, error out=w566:errorcluster)  [unwired: 1 out]
          n191 = VISA Write(VISA resource name=w564, write buffer=":tec?", error in (no error)=w566) -> (VISA resource name out=w563:refnum<visa-resource-name>, error out=w565:errorcluster)  [unwired: 1 out]
          n192 = VISA Read(VISA resource name=w563, byte count=u32 15, error in (no error)=w565) -> (VISA resource name out=w568:refnum<visa-resource-name>, read buffer=w558:string, error out=w567:errorcluster)  [unwired: 1 out]
          n193 = String Subset(string=w558, length (rest)=8 ("offset (0)")) -> (substring=w560:string)  [unwired: 1 in]
          n194 = Equal?(x=w560, y=":TEC OFF") -> (x = y?=w555:bool)
          n195 = Not(x=w555) -> (.not. x?=w554:bool)
          n196 = Bundle By Name(cluster=w557, "OnLine TEC"=w554) -> (w556:T2)
        }
        frame "On Line LD" {
          n197 = VISA Write(VISA resource name=w590, write buffer=w591, error in (no error)=w589) -> (VISA resource name out=w583:refnum<visa-resource-name>, error out=w585:errorcluster)  [unwired: 1 out]
          n198 = VISA Write(VISA resource name=w583, write buffer=":laser?", error in (no error)=w585) -> (VISA resource name out=w582:refnum<visa-resource-name>, error out=w584:errorcluster)  [unwired: 1 out]
          n199 = VISA Read(VISA resource name=w582, byte count=u32 15, error in (no error)=w584) -> (VISA resource name out=w587:refnum<visa-resource-name>, read buffer=w577:string, error out=w586:errorcluster)  [unwired: 1 out]
          n200 = String Subset(string=w577, length (rest)=10 ("offset (0)")) -> (substring=w579:string)  [unwired: 1 in]
          n201 = Equal?(x=w579, y=":LASER OFF") -> (x = y?=w574:bool)
          n202 = Not(x=w574) -> (.not. x?=w573:bool)
          n203 = Bundle By Name(cluster=w576, "OnLine LD"=w573) -> (w575:T2)
        }
        frame "Off Line TEC" {
          n204 = VISA Write(VISA resource name=w609, write buffer=w610, error in (no error)=w608) -> (VISA resource name out=w602:refnum<visa-resource-name>, error out=w604:errorcluster)  [unwired: 1 out]
          n205 = VISA Write(VISA resource name=w602, write buffer=":tec?", error in (no error)=w604) -> (VISA resource name out=w601:refnum<visa-resource-name>, error out=w603:errorcluster)  [unwired: 1 out]
          n206 = VISA Read(VISA resource name=w601, byte count=u32 15, error in (no error)=w603) -> (VISA resource name out=w606:refnum<visa-resource-name>, read buffer=w596:string, error out=w605:errorcluster)  [unwired: 1 out]
          n207 = String Subset(string=w596, length (rest)=8 ("offset (0)")) -> (substring=w598:string)  [unwired: 1 in]
          n208 = Equal?(x=w598, y=":TEC OFF") -> (x = y?=w593:bool)
          n209 = Not(x=w593) -> (.not. x?=w592:bool)
          n210 = Bundle By Name(cluster=w595, "OffLine TEC"=w592) -> (w594:T2)
        }
        frame "Off Line LD" {
          n211 = VISA Write(VISA resource name=w628, write buffer=w629, error in (no error)=w627) -> (VISA resource name out=w621:refnum<visa-resource-name>, error out=w623:errorcluster)  [unwired: 1 out]
          n212 = VISA Write(VISA resource name=w621, write buffer=":laser?", error in (no error)=w623) -> (VISA resource name out=w620:refnum<visa-resource-name>, error out=w622:errorcluster)  [unwired: 1 out]
          n213 = VISA Read(VISA resource name=w620, byte count=u32 15, error in (no error)=w622) -> (VISA resource name out=w625:refnum<visa-resource-name>, read buffer=w615:string, error out=w624:errorcluster)  [unwired: 1 out]
          n214 = String Subset(string=w615, length (rest)=10 ("offset (0)")) -> (substring=w617:string)  [unwired: 1 in]
          n215 = Equal?(x=w617, y=":LASER OFF") -> (x = y?=w612:bool)
          n216 = Not(x=w612) -> (.not. x?=w611:bool)
          n217 = Bundle By Name(cluster=w614, "OffLine LD"=w611) -> (w613:T2)
        }
        frame "Etalon TEC" {
          n218 = VISA Write(VISA resource name=w647, write buffer=w648, error in (no error)=w646) -> (VISA resource name out=w640:refnum<visa-resource-name>, error out=w642:errorcluster)  [unwired: 1 out]
          n219 = VISA Write(VISA resource name=w640, write buffer=":tec?", error in (no error)=w642) -> (VISA resource name out=w639:refnum<visa-resource-name>, error out=w641:errorcluster)  [unwired: 1 out]
          n220 = VISA Read(VISA resource name=w639, byte count=u32 15, error in (no error)=w641) -> (VISA resource name out=w644:refnum<visa-resource-name>, read buffer=w634:string, error out=w643:errorcluster)  [unwired: 1 out]
          n221 = String Subset(string=w634, length (rest)=8 ("offset (0)")) -> (substring=w636:string)  [unwired: 1 in]
          n222 = Equal?(x=w636, y=":TEC OFF") -> (x = y?=w631:bool)
          n223 = Not(x=w631) -> (.not. x?=w630:bool)
          n224 = Bundle By Name(cluster=w633, "Etalon TEC"=w630) -> (w632:T2)
        }
        frame "TSOA TEC" {
          n225 = VISA Write(VISA resource name=w666, write buffer=w667, error in (no error)=w665) -> (VISA resource name out=w659:refnum<visa-resource-name>, error out=w661:errorcluster)  [unwired: 1 out]
          n226 = VISA Write(VISA resource name=w659, write buffer=":tec?", error in (no error)=w661) -> (VISA resource name out=w658:refnum<visa-resource-name>, error out=w660:errorcluster)  [unwired: 1 out]
          n227 = VISA Read(VISA resource name=w658, byte count=u32 15, error in (no error)=w660) -> (VISA resource name out=w663:refnum<visa-resource-name>, read buffer=w653:string, error out=w662:errorcluster)  [unwired: 1 out]
          n228 = String Subset(string=w653, length (rest)=8 ("offset (0)")) -> (substring=w655:string)  [unwired: 1 in]
          n229 = Equal?(x=w655, y=":TEC OFF") -> (x = y?=w650:bool)
          n230 = Not(x=w650) -> (.not. x?=w649:bool)
          n231 = Bundle By Name(cluster=w652, "TSOA TEC"=w649) -> (w651:T2)
        }
      }
    }
    frame "Set_Limits" {
    }
    frame "Read_Limits" {
    }
    frame "Enable_Status" {
    }
    frame "Read_Status" {
      # "Read the on/off status, TEC set and actual temperatures and laser diode set and actual current and updates the front panel"
      n232 = for {
        tunnel: w687 -> [w695] mode=indexing
        tunnel: w686 -> [w696]
        tunnel: [w691] -> w682
        tunnel: w683 -> [w692]
        tunnel: [w693] -> w684
        shift-right: [w690] -> w680
        shift-left: w681 -> [w697]
        shift-right: [w689] -> _
        shift-left: w685 -> [w694]
        i -> [w698]
        n233 = case shown="2" w698 {
          tunnel: w697 -> [w711 w753 w789 w831 w867 w906]
          tunnel: w692 -> [w714 w756 w792 w834 w870 w909]
          tunnel: w696 -> [w713 w755 w791 w833 w869 w908]
          tunnel: w695 -> [w712 w754 w790 w832 w868 w907]
          tunnel: w694 -> [w708 w749 w785 w827 w863 w902]
          tunnel: [w703 w744 w780 w822 w858 w897] -> w693
          tunnel: [w702 w743 w779 w821 w857 w896] -> w691
          tunnel: [w700 w738 w778 w817 w855 w894] -> w690
          tunnel: [w701 w739 w777 w816 w856 w895] -> w689
          frame 0, Default {
            n234 = Concatenate Strings(w712, ";:tec?" ("write buffer")) -> (w734:string)
            n235 = Concatenate Strings(w712, ";:temp:set?" ("write buffer")) -> (w721:string)
            n236 = Concatenate Strings(w712, ";:temp:act?" ("write buffer")) -> (w716:string)
            n237 = VISA Write(VISA resource name=w714, write buffer=w734, error in (no error)=w713) -> (VISA resource name out=w735:refnum<visa-resource-name>, error out=w736:errorcluster)  [unwired: 1 out]
            n238 = VISA Read(VISA resource name=w735, byte count=u32 30, error in (no error)=w736) -> (VISA resource name out=w725:refnum<visa-resource-name>, read buffer=w729:string, error out=w724:errorcluster)  [unwired: 1 out]
            n239 = String Subset(string=w729, length (rest)=7 ("offset (0)")) -> (substring=w731:string)  [unwired: 1 in]
            n240 = VISA Write(VISA resource name=w725, write buffer=w721, error in (no error)=w724) -> (VISA resource name out=w726:refnum<visa-resource-name>, error out=w727:errorcluster)  [unwired: 1 out]
            n241 = Equal?(x=w731, y=":TEC ON") -> (x = y?=w699:bool)
            n242 = VISA Read(VISA resource name=w726, byte count=u32 30, error in (no error)=w727) -> (VISA resource name out=w717:refnum<visa-resource-name>, read buffer=w709:string, error out=w718:errorcluster)  [unwired: 1 out]
            n243 = Fract/Exp String To Number(string=w709, offset=10) -> (number=w704:dbl)  [unwired: 2 in, 1 out]
            n244 = VISA Write(VISA resource name=w717, write buffer=w716, error in (no error)=w718) -> (VISA resource name out=w719:refnum<visa-resource-name>, error out=w715:errorcluster)  [unwired: 1 out]
            n245 = VISA Read(VISA resource name=w719, byte count=u32 30, error in (no error)=w715) -> (VISA resource name out=w703:refnum<visa-resource-name>, read buffer=w706:string, error out=w702:errorcluster)  [unwired: 1 out]
            n246 = Fract/Exp String To Number(string=w706, offset=10) -> (number=w705:dbl)  [unwired: 2 in, 1 out]
            n247 = Bundle By Name(cluster=w708, "OnLineTEC"=w704) -> (w701:T3)
            n248 = Bundle By Name(cluster=w711, "OnLineTEC"=w705, "OnLine TEC"=w699, "Pro8000"=w699) -> (w700:T2)
            n249 = local write "Readings"(w700) -> ()
            n250 = local write "Settings"(w701) -> ()
          }
          frame 1 {
            n251 = Concatenate Strings(w754, ";:laser?" ("write buffer")) -> (w773:string)
            n252 = Concatenate Strings(w754, ";:ild:set?" ("write buffer")) -> (w763:string)
            n253 = Concatenate Strings(w754, ";:ild:act?" ("write buffer")) -> (w758:string)
            n254 = VISA Write(VISA resource name=w756, write buffer=w773, error in (no error)=w755) -> (VISA resource name out=w774:refnum<visa-resource-name>, error out=w775:errorcluster)  [unwired: 1 out]
            n255 = VISA Read(VISA resource name=w774, byte count=u32 30, error in (no error)=w775) -> (VISA resource name out=w765:refnum<visa-resource-name>, read buffer=w769:string, error out=w764:errorcluster)  [unwired: 1 out]
            n256 = String Subset(string=w769, length (rest)=9 ("offset (0)")) -> (substring=w771:string)  [unwired: 1 in]
            n257 = VISA Write(VISA resource name=w765, write buffer=w763, error in (no error)=w764) -> (VISA resource name out=w766:refnum<visa-resource-name>, error out=w767:errorcluster)  [unwired: 1 out]
            n258 = Equal?(x=w771, y=":LASER ON") -> (x = y?=w752:bool)
            n259 = VISA Read(VISA resource name=w766, byte count=u32 30, error in (no error)=w767) -> (VISA resource name out=w759:refnum<visa-resource-name>, read buffer=w750:string, error out=w760:errorcluster)  [unwired: 1 out]
            n260 = Fract/Exp String To Number(string=w750, offset=9) -> (number=w745:dbl)  [unwired: 2 in, 1 out]
            n261 = VISA Write(VISA resource name=w759, write buffer=w758, error in (no error)=w760) -> (VISA resource name out=w761:refnum<visa-resource-name>, error out=w757:errorcluster)  [unwired: 1 out]
            n262 = VISA Read(VISA resource name=w761, byte count=u32 30, error in (no error)=w757) -> (VISA resource name out=w744:refnum<visa-resource-name>, read buffer=w747:string, error out=w743:errorcluster)  [unwired: 1 out]
            n263 = Fract/Exp String To Number(string=w747, offset=9) -> (number=w746:dbl)  [unwired: 2 in, 1 out]
            n264 = Bundle By Name(cluster=w749, "OnLineLD"=w745) -> (w739:T3)
            n265 = Bundle By Name(cluster=w753, "OnLineLD"=w746, "OnLine LD"=w752) -> (w738:T2)
            n266 = local write "Readings"(w738) -> ()
            n267 = local write "Settings"(w739) -> ()
          }
          frame 2 {
            n268 = Concatenate Strings(w790, ";:tec?" ("write buffer")) -> (w812:string)
            n269 = Concatenate Strings(w790, ";:temp:set?" ("write buffer")) -> (w799:string)
            n270 = Concatenate Strings(w790, ";:temp:act?" ("write buffer")) -> (w794:string)
            n271 = VISA Write(VISA resource name=w792, write buffer=w812, error in (no error)=w791) -> (VISA resource name out=w813:refnum<visa-resource-name>, error out=w814:errorcluster)  [unwired: 1 out]
            n272 = VISA Read(VISA resource name=w813, byte count=u32 30, error in (no error)=w814) -> (VISA resource name out=w803:refnum<visa-resource-name>, read buffer=w807:string, error out=w802:errorcluster)  [unwired: 1 out]
            n273 = String Subset(string=w807, length (rest)=7 ("offset (0)")) -> (substring=w809:string)  [unwired: 1 in]
            n274 = VISA Write(VISA resource name=w803, write buffer=w799, error in (no error)=w802) -> (VISA resource name out=w804:refnum<visa-resource-name>, error out=w805:errorcluster)  [unwired: 1 out]
            n275 = Equal?(x=w809, y=":TEC ON") -> (x = y?=w788:bool)
            n276 = VISA Read(VISA resource name=w804, byte count=u32 30, error in (no error)=w805) -> (VISA resource name out=w795:refnum<visa-resource-name>, read buffer=w786:string, error out=w796:errorcluster)  [unwired: 1 out]
            n277 = Fract/Exp String To Number(string=w786, offset=10) -> (number=w781:dbl)  [unwired: 2 in, 1 out]
            n278 = VISA Write(VISA resource name=w795, write buffer=w794, error in (no error)=w796) -> (VISA resource name out=w797:refnum<visa-resource-name>, error out=w793:errorcluster)  [unwired: 1 out]
            n279 = VISA Read(VISA resource name=w797, byte count=u32 30, error in (no error)=w793) -> (VISA resource name out=w780:refnum<visa-resource-name>, read buffer=w783:string, error out=w779:errorcluster)  [unwired: 1 out]
            n280 = Fract/Exp String To Number(string=w783, offset=10) -> (number=w782:dbl)  [unwired: 2 in, 1 out]
            n281 = Bundle By Name(cluster=w785, "OffLineTEC"=w781) -> (w777:T3)
            n282 = Bundle By Name(cluster=w789, "OffLineTEC"=w782, "OffLine TEC"=w788) -> (w778:T2)
            n283 = local write "Readings"(w778) -> ()
            n284 = local write "Settings"(w777) -> ()
          }
          frame 3 {
            n285 = Concatenate Strings(w832, ";:laser?" ("write buffer")) -> (w851:string)
            n286 = Concatenate Strings(w832, ";:ild:set?" ("write buffer")) -> (w841:string)
            n287 = Concatenate Strings(w832, ";:ild:act?" ("write buffer")) -> (w836:string)
            n288 = VISA Write(VISA resource name=w834, write buffer=w851, error in (no error)=w833) -> (VISA resource name out=w852:refnum<visa-resource-name>, error out=w853:errorcluster)  [unwired: 1 out]
            n289 = VISA Read(VISA resource name=w852, byte count=u32 30, error in (no error)=w853) -> (VISA resource name out=w843:refnum<visa-resource-name>, read buffer=w847:string, error out=w842:errorcluster)  [unwired: 1 out]
            n290 = String Subset(string=w847, length (rest)=9 ("offset (0)")) -> (substring=w849:string)  [unwired: 1 in]
            n291 = VISA Write(VISA resource name=w843, write buffer=w841, error in (no error)=w842) -> (VISA resource name out=w844:refnum<visa-resource-name>, error out=w845:errorcluster)  [unwired: 1 out]
            n292 = Equal?(x=w849, y=":LASER ON") -> (x = y?=w830:bool)
            n293 = VISA Read(VISA resource name=w844, byte count=u32 30, error in (no error)=w845) -> (VISA resource name out=w837:refnum<visa-resource-name>, read buffer=w828:string, error out=w838:errorcluster)  [unwired: 1 out]
            n294 = Fract/Exp String To Number(string=w828, offset=9) -> (number=w823:dbl)  [unwired: 2 in, 1 out]
            n295 = VISA Write(VISA resource name=w837, write buffer=w836, error in (no error)=w838) -> (VISA resource name out=w839:refnum<visa-resource-name>, error out=w835:errorcluster)  [unwired: 1 out]
            n296 = VISA Read(VISA resource name=w839, byte count=u32 30, error in (no error)=w835) -> (VISA resource name out=w822:refnum<visa-resource-name>, read buffer=w825:string, error out=w821:errorcluster)  [unwired: 1 out]
            n297 = Fract/Exp String To Number(string=w825, offset=9) -> (number=w824:dbl)  [unwired: 2 in, 1 out]
            n298 = Bundle By Name(cluster=w827, "OffLineLD"=w823) -> (w816:T3)
            n299 = Bundle By Name(cluster=w831, "OffLineLD"=w824, "OffLine LD"=w830) -> (w817:T2)
            n300 = local write "Readings"(w817) -> ()
            n301 = local write "Settings"(w816) -> ()
          }
          frame 4 {
            n302 = Concatenate Strings(w868, ";:tec?" ("write buffer")) -> (w890:string)
            n303 = Concatenate Strings(w868, ";:temp:set?" ("write buffer")) -> (w877:string)
            n304 = Concatenate Strings(w868, ";:temp:act?" ("write buffer")) -> (w872:string)
            n305 = VISA Write(VISA resource name=w870, write buffer=w890, error in (no error)=w869) -> (VISA resource name out=w891:refnum<visa-resource-name>, error out=w892:errorcluster)  [unwired: 1 out]
            n306 = VISA Read(VISA resource name=w891, byte count=u32 30, error in (no error)=w892) -> (VISA resource name out=w881:refnum<visa-resource-name>, read buffer=w885:string, error out=w880:errorcluster)  [unwired: 1 out]
            n307 = String Subset(string=w885, length (rest)=7 ("offset (0)")) -> (substring=w887:string)  [unwired: 1 in]
            n308 = VISA Write(VISA resource name=w881, write buffer=w877, error in (no error)=w880) -> (VISA resource name out=w882:refnum<visa-resource-name>, error out=w883:errorcluster)  [unwired: 1 out]
            n309 = Equal?(x=w887, y=":TEC ON") -> (x = y?=w866:bool)
            n310 = VISA Read(VISA resource name=w882, byte count=u32 30, error in (no error)=w883) -> (VISA resource name out=w873:refnum<visa-resource-name>, read buffer=w864:string, error out=w874:errorcluster)  [unwired: 1 out]
            n311 = Fract/Exp String To Number(string=w864, offset=10) -> (number=w859:dbl)  [unwired: 2 in, 1 out]
            n312 = VISA Write(VISA resource name=w873, write buffer=w872, error in (no error)=w874) -> (VISA resource name out=w875:refnum<visa-resource-name>, error out=w871:errorcluster)  [unwired: 1 out]
            n313 = VISA Read(VISA resource name=w875, byte count=u32 30, error in (no error)=w871) -> (VISA resource name out=w858:refnum<visa-resource-name>, read buffer=w861:string, error out=w857:errorcluster)  [unwired: 1 out]
            n314 = Fract/Exp String To Number(string=w861, offset=10) -> (number=w860:dbl)  [unwired: 2 in, 1 out]
            n315 = Bundle By Name(cluster=w863, "EtalonTEC"=w859) -> (w856:T3)
            n316 = Bundle By Name(cluster=w867, "EtalonTEC"=w860, "Etalon TEC"=w866) -> (w855:T2)
            n317 = local write "Readings"(w855) -> ()
            n318 = local write "Settings"(w856) -> ()
          }
          frame 5 {
            n319 = Concatenate Strings(w907, ";:tec?" ("write buffer")) -> (w929:string)
            n320 = Concatenate Strings(w907, ";:temp:set?" ("write buffer")) -> (w916:string)
            n321 = Concatenate Strings(w907, ";:temp:act?" ("write buffer")) -> (w911:string)
            n322 = VISA Write(VISA resource name=w909, write buffer=w929, error in (no error)=w908) -> (VISA resource name out=w930:refnum<visa-resource-name>, error out=w931:errorcluster)  [unwired: 1 out]
            n323 = VISA Read(VISA resource name=w930, byte count=u32 30, error in (no error)=w931) -> (VISA resource name out=w920:refnum<visa-resource-name>, read buffer=w924:string, error out=w919:errorcluster)  [unwired: 1 out]
            n324 = String Subset(string=w924, length (rest)=7 ("offset (0)")) -> (substring=w926:string)  [unwired: 1 in]
            n325 = VISA Write(VISA resource name=w920, write buffer=w916, error in (no error)=w919) -> (VISA resource name out=w921:refnum<visa-resource-name>, error out=w922:errorcluster)  [unwired: 1 out]
            n326 = Equal?(x=w926, y=":TEC ON") -> (x = y?=w905:bool)
            n327 = VISA Read(VISA resource name=w921, byte count=u32 30, error in (no error)=w922) -> (VISA resource name out=w912:refnum<visa-resource-name>, read buffer=w903:string, error out=w913:errorcluster)  [unwired: 1 out]
            n328 = Fract/Exp String To Number(string=w903, offset=10) -> (number=w898:dbl)  [unwired: 2 in, 1 out]
            n329 = VISA Write(VISA resource name=w912, write buffer=w911, error in (no error)=w913) -> (VISA resource name out=w914:refnum<visa-resource-name>, error out=w910:errorcluster)  [unwired: 1 out]
            n330 = VISA Read(VISA resource name=w914, byte count=u32 30, error in (no error)=w910) -> (VISA resource name out=w897:refnum<visa-resource-name>, read buffer=w900:string, error out=w896:errorcluster)  [unwired: 1 out]
            n331 = Fract/Exp String To Number(string=w900, offset=10) -> (number=w899:dbl)  [unwired: 2 in, 1 out]
            n332 = Bundle By Name(cluster=w902, "TSOA-TEC"=w898) -> (w895:T3)
            n333 = Bundle By Name(cluster=w906, "TSOA-TEC"=w899, "TSOA TEC"=w905) -> (w894:T2)
            n334 = local write "Readings"(w894) -> ()
            n335 = local write "Settings"(w895) -> ()
          }
        }
      }
    }
  }
  "error out" <- w15
  "Device Out" <- w11
  "Response" <- w10
  "Readings" <- w1
